vi "Go Home Sub_VI.vi"(8 "error in (no error)":errorcluster, 9 "stop":bool, 10 "Homing Freq":dbl format="%#_13g", 11 "Homing Duty %":dbl format="%#_13g") -> (0 "error out":errorcluster, 2 "Motor Status out":T2 {"Y Velocity (mm/s)" format="%#_3g"; "X Velocity (mm/s)" format="%#_3g"; "Homing Duty %" format="%#_13g"; "Homing Freq" format="%#_13g"})   [LabVIEW 2017]
uses:
  Go Home State type def.ctl
panel:
  # "Go Home Sub_VI.vi instructions:\n1. Enter Homing Duty Cycle % for X axis and Homing Frequency for Y axis\n2. Run VI, XY axes will move to home position and stop automatically\n\nRecommended values:\nFrequency = 20000\nDuty % = 80"
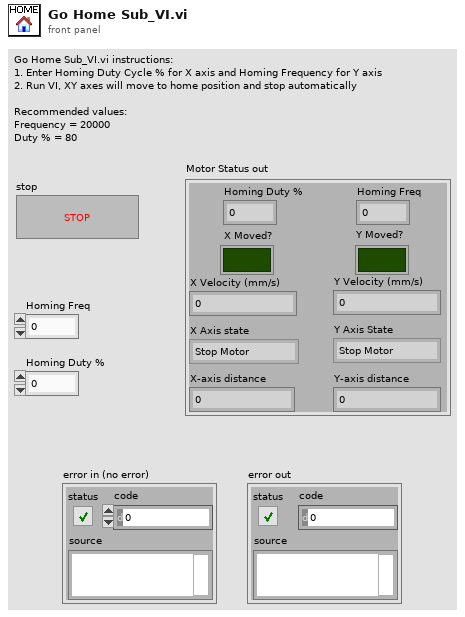
[diagram p1: front panel]
types:
  T1 = typedef "Go Home State type def.ctl" = enum16{"Stop Motor", "Read Input", "Drive Motor"}
  T2 = cluster{"Homing Freq":dbl, "Homing Duty %":dbl, "X Moved?":bool, "Y Moved?":bool, "X Axis state":T1, "Y Axis State":T1, "X-axis distance":dbl, "X Velocity (mm/s)":dbl, "Y-axis distance":dbl, "Y Velocity (mm/s)":dbl}
  T3 = typedef "Encoder Cluster.ctl" = cluster{"Y-axis rev count":dbl, "Y-axis distance":dbl, "X-axis rev count":dbl, "X-axis distance":dbl, "Y-axis direction":T4, "X-axis direction":T4, "X-counter val":i32, "Y-counter val":i32}
  T4 = typedef "Encoder Count Direction Enum.ctl" = enum16{"Counting Up", "Counting Down"}
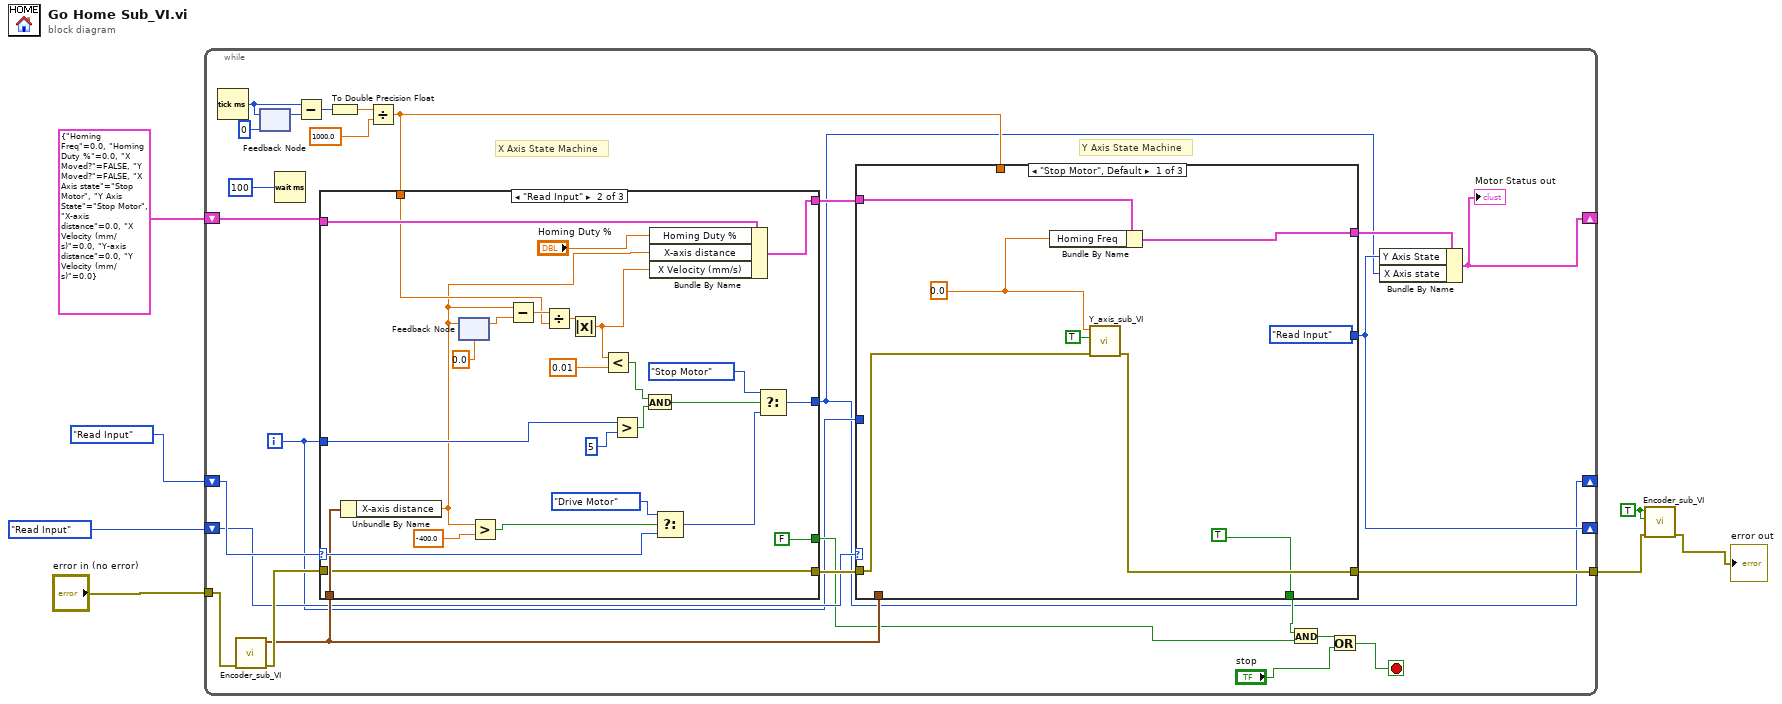
[diagram p0: block diagram]
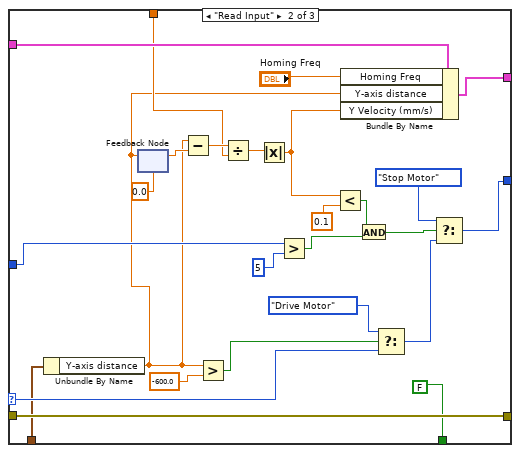
[diagram p2: hidden frame]
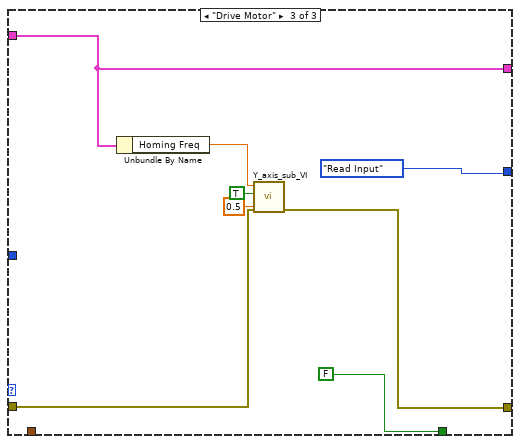
[diagram p3: hidden frame]
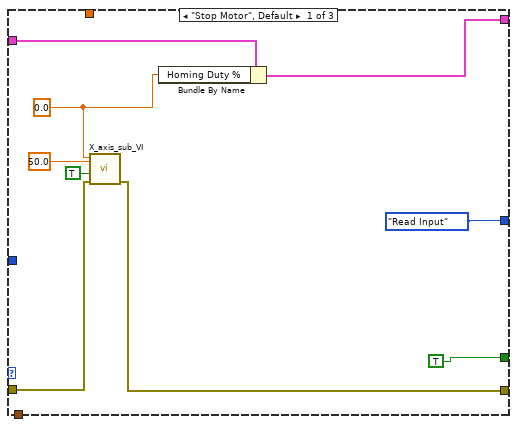
[diagram p4: hidden frame]
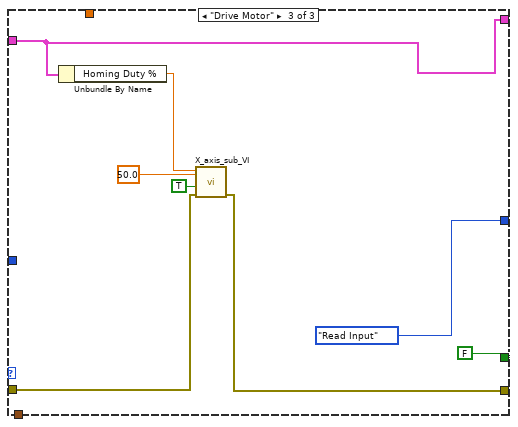
[diagram p5: hidden frame]
diagram:
  w1 = TRUE ("Reset X Counter")
  n1 = while {
    tunnel: "error in (no error)" -> [w33]
    tunnel: [w30] -> w3
    shift-right: [w9] -> _
    shift-left: Go_Home_State_type_def."Read Input" ("Enum 2") -> [w32]
    shift-right: [w11] -> _
    shift-left: T2 {"Homing Freq"=0.0, "Homing Duty %"=0.0, "X Moved?"=FALSE, "Y Moved?"=FALSE, "X Axis state"=enum."Stop Motor", "Y Axis State"=enum."Stop Motor", "X-axis distance"=0.0, "X Velocity (mm/s)"=0.0, "Y-axis distance"=0.0, "Y Velocity (mm/s)"=0.0} ("Motor Status out 2") -> [w34]
    shift-right: [w10] -> _
    shift-left: Go_Home_State_type_def."Read Input" ("Enum") -> [w26]
    i -> [w13]
    stop <- w14 stop-if-true
    # "Y Axis State Machine"
    # "X Axis State Machine"
    n2 = Tick Count (ms)() -> (millisecond timer value=w22:u32)
    n3 = call "Encoder_sub_VI.vi"("error in (no error)"=w33) -> ("error out"=w28:errorcluster, "Encoder Output"=w27:T3)  [unwired: 9 in]
    n4 = feedback-in #1(w22) -> ()
    n5 = feedback #1(u32 0 ("millisecond timer value")) -> (w21:u32)
    n6 = Wait (ms)(milliseconds to wait=u32 100) -> ()  [unwired: 1 out]
    n7 = Subtract(x=w22, y=w21) -> (x-y=w20:u32)
    n8 = To Double Precision Float(number=w20) -> (double precision float=w19:dbl)
    n9 = Divide(x=w19, y=1000.0) -> (x/y=w23:dbl)
    n10 = case shown="\"Read Input\"" w32 {
      selector: w32 -> [_ w108 _]
      tunnel: w34 -> [w85 w103 w112]
      tunnel: [w84 w110 w112] -> w31
      tunnel: [Go_Home_State_type_def."Read Input" w104 Go_Home_State_type_def."Read Input"] -> w9
      tunnel: w28 -> [w83 w98 w117]
      tunnel: [w78 w98 w116] -> w29
      tunnel: [TRUE FALSE FALSE] -> w17
      tunnel: w27 -> [_ w106 _]
      tunnel: w23 -> [_ w89 _]
      tunnel: w13 -> [_ w97 _]
      frame "Stop Motor", Default {
        w82 = 0.0
        n11 = call "X_axis_sub_VI.vi"("error in (no error)"=w83, "FWD/RVS"=TRUE, "Frequency"=50.0, "Duty Cycle %"=w82) -> ("error out"=w78:errorcluster)  [unwired: 7 in]
        n12 = Bundle By Name(cluster=w85, "Homing Duty %"=w82) -> (w84:T2)
      }
      frame "Read Input" {
        n13 = Unbundle By Name(w106) -> ("X-axis distance"=w87:dbl)
        n14 = feedback #2(0.0 ("X-axis distance")) -> (w92:dbl)
        n15 = feedback-in #2(w87) -> ()
        n16 = Greater?(x=w87, y=-400.0) -> (0:w102:bool)
        n17 = Subtract(x=w87, y=w92) -> (x-y=w90:dbl)
        n18 = Divide(x=w90, y=w89) -> (x/y=w88:dbl)
        n19 = Absolute Value(x=w88) -> (abs(x)=w86:dbl)
        n20 = Less?(x=w86, y=0.01) -> (x < y?=w94:bool)
        n21 = Greater?(x=w97, y=5) -> (0:w95:bool)
        n22 = And(x=w94, y=w95) -> (x .and. y?=w93:bool)
        n23 = Bundle By Name(cluster=w103, "Homing Duty %"="Homing Duty %", "X-axis distance"=w87, "X Velocity (mm/s)"=w86) -> (w110:T2)
        n24 = Select(t=Go_Home_State_type_def."Drive Motor", s=w102, f=w108) -> (s? t:f=w101:T1)
        n25 = Select(t=Go_Home_State_type_def."Stop Motor", s=w93, f=w101) -> (s? t:f=w104:T1)
      }
      frame "Drive Motor" {
        n26 = Unbundle By Name(w112) -> ("Homing Duty %"=w115:dbl)
        n27 = call "X_axis_sub_VI.vi"("error in (no error)"=w117, "FWD/RVS"=TRUE, "Frequency"=50.0, "Duty Cycle %"=w115) -> ("error out"=w116:errorcluster)  [unwired: 7 in]
      }
    }
    n28 = case shown="\"Stop Motor\", Default" w26 {
      selector: w26 -> [_ w66 _]
      tunnel: [w42 w68 w70] -> w12
      tunnel: [Go_Home_State_type_def."Read Input" w64 Go_Home_State_type_def."Read Input"] -> w10
      tunnel: w29 -> [w35 w61 w74]
      tunnel: [w41 w61 w73] -> w30
      tunnel: [TRUE FALSE FALSE ("stop")] -> w18
      tunnel: w31 -> [w36 w59 w70]
      tunnel: w27 -> [_ w60 _]
      tunnel: w23 -> [_ w49 _]
      tunnel: w13 -> [_ w45 _]
      frame "Stop Motor", Default {
        w40 = 0.0
        n29 = Bundle By Name(cluster=w36, "Homing Freq"=w40) -> (w42:T2)
        n30 = call "Y_axis_sub_VI.vi"("error in (no error)"=w35, "FWD/RVS"=TRUE, "Frequency"=w40) -> ("error out"=w41:errorcluster)  [unwired: 8 in]
      }
      frame "Read Input" {
        n31 = Unbundle By Name(w60) -> ("Y-axis distance"=w43:dbl)
        n32 = feedback #3(0.0 ("X-axis distance")) -> (w50:dbl)
        n33 = feedback-in #3(w43) -> ()
        n34 = Subtract(x=w43, y=w50) -> (x-y=w51:dbl)
        n35 = Greater?(x=w43, y=-600.0) -> (0:w57:bool)
        n36 = Divide(x=w51, y=w49) -> (x/y=w52:dbl)
        n37 = Absolute Value(x=w52) -> (abs(x)=w44:dbl)
        n38 = Greater?(x=w45, y=5) -> (0:w46:bool)
        n39 = Less?(x=w44, y=0.1) -> (x < y?=w54:bool)
        n40 = Bundle By Name(cluster=w59, "Homing Freq"="Homing Freq", "Y-axis distance"=w43, "Y Velocity (mm/s)"=w44) -> (w68:T2)
        n41 = And(x=w54, y=w46) -> (x .and. y?=w55:bool)
        n42 = Select(t=Go_Home_State_type_def."Drive Motor", s=w57, f=w66) -> (s? t:f=w58:T1)
        n43 = Select(t=Go_Home_State_type_def."Stop Motor", s=w55, f=w58) -> (s? t:f=w64:T1)
      }
      frame "Drive Motor" {
        n44 = Unbundle By Name(w70) -> ("Homing Freq"=w71:dbl)
        n45 = call "Y_axis_sub_VI.vi"("error in (no error)"=w74, "Duty Cycle"=0.5, "FWD/RVS"=TRUE, "Frequency"=w71) -> ("error out"=w73:errorcluster)  [unwired: 7 in]
      }
    }
    n46 = And(x=w18, y=w17) -> (x .and. y?=w16:bool)
    n47 = Or(x=w16, y="stop") -> (x .or. y?=w14:bool)
    n48 = Bundle By Name(cluster=w12, "Y Axis State"=w10, "X Axis state"=w9) -> (w11:T2)
    "Motor Status out" <- w11
  }
  n49 = call "Encoder_sub_VI.vi"("error in (no error)"=w3, "Reset Y Counter"=w1, "Reset X Counter"=w1) -> ("error out"=→"error out":errorcluster)  [unwired: 7 in, 1 out]
